vi "SQLSetStmAttr.vi"(4 "error in (no error)":errorcluster, 5 "AttributeValue":u32, 6 "AttributePosition":i32, 7 "InputHandle":i32) -> (0 "error out":errorcluster, 3 "OutputHandle":i32)   [LabVIEW 2011]
doc: "Configure la requête en fonction des paramètres d'entrée"
uses:
  Odbc32.dll
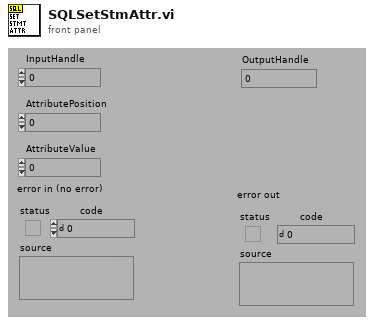
[diagram p1: front panel]
types:
  T1 = enum16{"NOPE", "SQL_HANDLE_ENV", "SQL_HANDLE_DBC", "SQL_HANDLE_STMT", "SQL_HANDLE_DESC"}
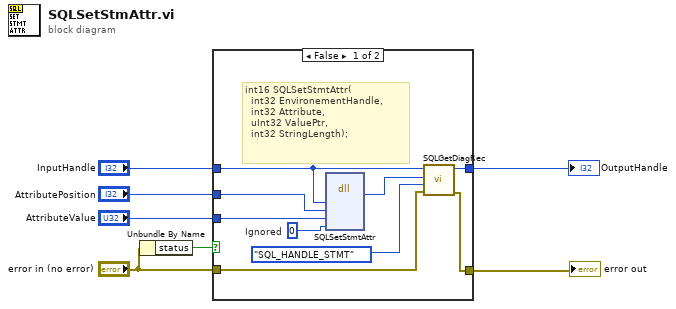
[diagram p0: block diagram]
diagram:
  n1 = Unbundle By Name("error in (no error)") -> ("status"=w1:bool)
  n2 = case shown="False" w1 {
    tunnel: "AttributePosition" -> [w16 _]
    tunnel: "AttributeValue" -> [w15 _]
    tunnel: [w13 w18] -> w5
    tunnel: "InputHandle" -> [w12 w18]
    tunnel: "error in (no error)" -> [w10 w17]
    tunnel: [w9 w17] -> w3
    frame False {
      w14 = 0  # Ignored
      # "int16 SQLSetStmtAttr(\n  int32 EnvironementHandle, \n  int32 Attribute, \n  uInt32 ValuePtr, \n  int32 StringLength);"
      n3 = dll-call lib="Odbc32.dll" fn="SQLSetStmtAttr"("EnvironementHandle"=w12, "Attribute"=w16, "ValuePtr"=w15, "StringLength"=w14) -> (w11:i16)  [unwired: 7 in, 2 out]
      n4 = call "SQLGetDiagRec.vi"("error in (no error)"=w10, "HandleType"=T1."SQL_HANDLE_STMT", "Status (SQL_SUCCESS=0)"=w11, "Input Handle"=w12) -> ("error out"=w9:errorcluster, "Output Handle"=w13:i32)  [unwired: 2 out]
    }
    frame True {
    }
  }
  "OutputHandle" <- w5
  "error out" <- w3
